vi "Projectile(with_SUB-VI).vi"() -> ()   [LabVIEW 2015]
panel:
  out "Range (m)":dbl format="%.3f"
  out "Time of Flight (s)":dbl format="%.3f"
  out "Max. Height (m)":dbl format="%.3f"
  in  "Theta (deg)":dbl
  in  "v (m/s)":dbl
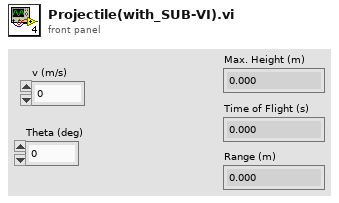
[diagram p1: front panel]
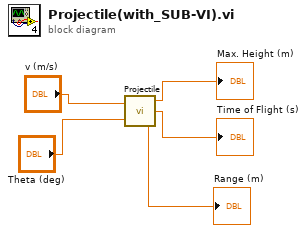
[diagram p0: block diagram]
diagram:
  n1 = call "Projectile.vi"("v (m/s)"="v (m/s)", "Theta (deg)"="Theta (deg)") -> ("Max. Height (m)"=→"Max. Height (m)":dbl, "Time of Flight (sec)"=→"Time of Flight (s)":dbl, "Range (m)"=→"Range (m)":dbl)
